vi "GetSpeedWithCache.vi"(9 "pulse positions":T2, 10 "channel":T3, 11 "Map":T1) -> (2 "pulse position data":dbl[](array[numeric]), 3 "speed (RPM)":dbl)   [LabVIEW 2017, in "AnalysisHelper.lvlib"]
uses:
  <vilib>/addons/InsightCM/Utilities/Analysis/Shared/AnalysisHelper.lvlib
  <vilib>/addons/InsightCM/Utilities/Analysis/Shared/controls/Channel.ctl
  <vilib>/addons/InsightCM/Utilities/Analysis/Shared/controls/SpeedType.ctl
  <vilib>/addons/InsightCM/Utilities/Analysis/Shared/controls/Feature.ctl
  <vilib>/addons/InsightCM/Utilities/Analysis/Shared/controls/AmplitudeScale.ctl
  <vilib>/addons/InsightCM/Utilities/Analysis/Shared/controls/PulsePositions.ctl
  <vilib>/addons/PointValueMap/controls/PointMap.ctl
  <vilib>/addons/InsightCM/Utilities/Analysis/Shared/controls/SpeedCacheOps.ctl
  <vilib>/addons/PointValueMap/subVIs/Point_Read_double.vi
  <vilib>/addons/PointValueMap/PointValueMap.lvlib
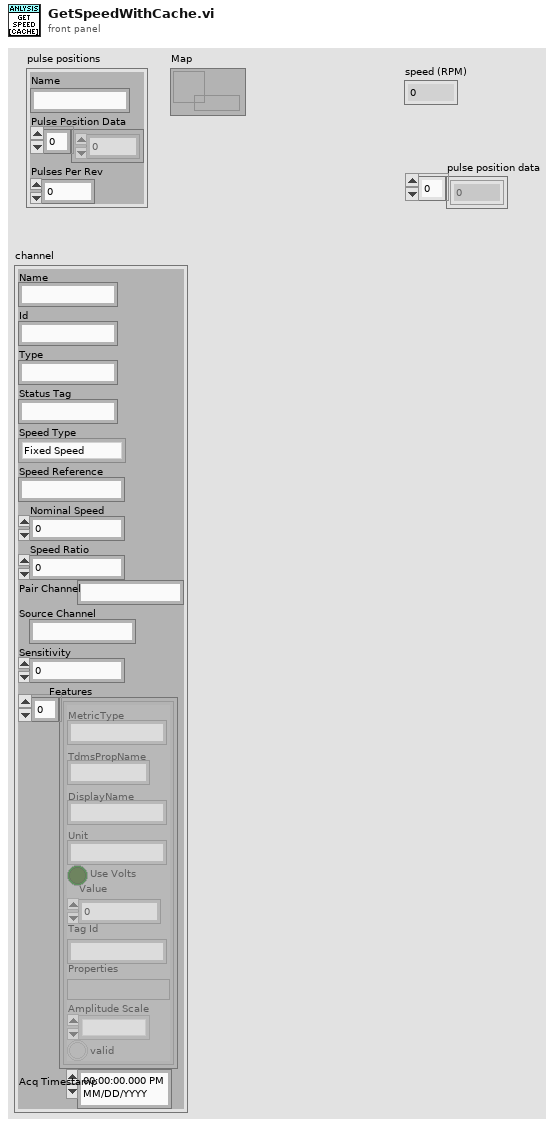
[diagram p1: front panel]
types:
  T1 = typedef "PointValueMap.lvlib/PointMap.ctl" = refnum<data-value>
  T2 = typedef "AnalysisHelper.lvlib/PulsePositions.ctl" = cluster{"Name":string, "Pulse Position Data":dbl[], "Pulses Per Rev":i32}
  T3 = typedef "AnalysisHelper.lvlib/Channel.ctl" = cluster{"Name":string, "Id":string, "Type":string, "Status Tag":string, "Speed Type":T4, "Speed Reference":string, "Nominal Speed":dbl, "Speed Ratio":dbl, "Pair Channel":string, "Source Channel":string, "Sensitivity":dbl, "Features":T5[], "Acq Timestamp":timestamp}
  T4 = typedef "AnalysisHelper.lvlib/SpeedType.ctl" = enum16{"Fixed Speed", "Tachometer", "From Map"}
  T5 = typedef "AnalysisHelper.lvlib/Feature.ctl" = cluster{"MetricType":string, "TdmsPropName":string, "DisplayName":string, "Unit":string, "Use Volts":bool, "Value":dbl, "Tag Id":string, "Properties":variant, "Amplitude Scale":T6, "valid":bool}
  T6 = typedef "AnalysisHelper.lvlib/AmplitudeScale.ctl" = enum16{"rms", "peak", "pk-pk"}
  T7 = typedef "AnalysisHelper.lvlib/SpeedCacheOps.ctl" = enum16{"Init", "GetSpeed"}
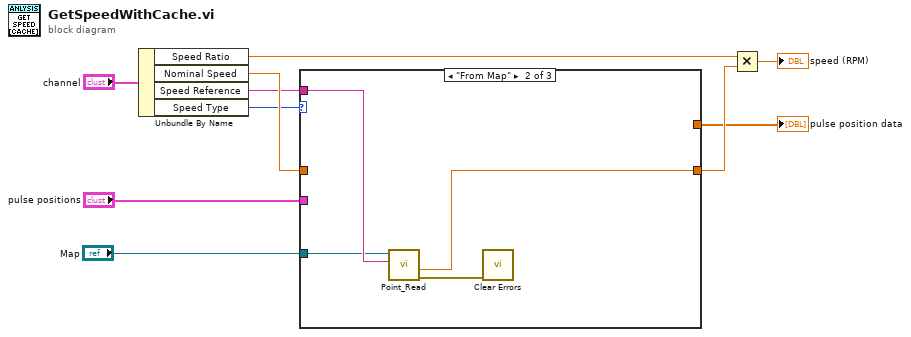
[diagram p0: block diagram]
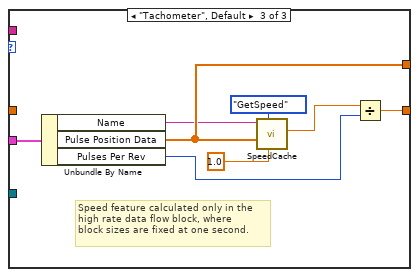
[diagram p3: hidden frame]
diagram:
  n1 = Unbundle By Name("channel") -> ("Speed Ratio"=w5:dbl, "Nominal Speed"=w6:dbl, "Speed Reference"=w2:string, "Speed Type"=w3:T4)
  n2 = case shown="\"From Map\"" w3 {
    tunnel: [w11 w13 w20] -> w7
    tunnel: "pulse positions" -> [_ _ w23]
    tunnel: w6 -> [w11 _ _]
    tunnel: [_ _ w22] -> w4
    tunnel: "Map" -> [_ w14 _]
    tunnel: w2 -> [_ w15 _]
    frame "Fixed Speed" {
    }
    frame "From Map" {
      n3 = call-poly <vilib>:"Point_Read.vi"("Tag"=w15, "Map"=w14) -> ("Error Out"=w12:errorcluster, "Value"=w13:dbl)  [unwired: 4 in, 4 out]
      n4 = call <vilib>:"Clear Errors.vi"("error in (no error)"=w12) -> ()  [unwired: 5 in, 2 out]
    }
    frame "Tachometer", Default {
      # "Speed feature calculated only in the \nhigh rate data flow block, where \nblock sizes are fixed at one second."
      n5 = Unbundle By Name(w23) -> ("Name"=w19:string, "Pulse Position Data"=w22:dbl[], "Pulses Per Rev"=w21:i32)
      n6 = call <vilib>:"SpeedCache.vi"("size of this data block"=1.0, "operation"=SpeedCacheOps."GetSpeed", "pulse position data"=w22, "channel"=w19) -> ("speed (RPM)"=w16:dbl)  [unwired: 5 in, 2 out]
      n7 = Divide(x=w16, y=w21) -> (x/y=w20:dbl)
    }
  }
  "pulse position data" <- w4
  n8 = Multiply(x=w5, y=w7) -> (x*y=→"speed (RPM)":dbl)
